vi "Config_flotas_baja_velocidad.vi"(11 "file path (dialog if empty)":path) -> (0 "Radios ruedas":dbl[](array[numeric]), 1 "Distancias generales":dbl[](array[numeric]), 2 "Puntos medios de las ventanas":dbl[][](array[numeric]), 3 "Distancia de acelerómetros":dbl[](array[numeric]), 5 "Distacias y medidas de dispositivos":bool=TRUE, 7 "Series_flota":string[](array[string]))   [LabVIEW 2015]
panel:
  out "text":string
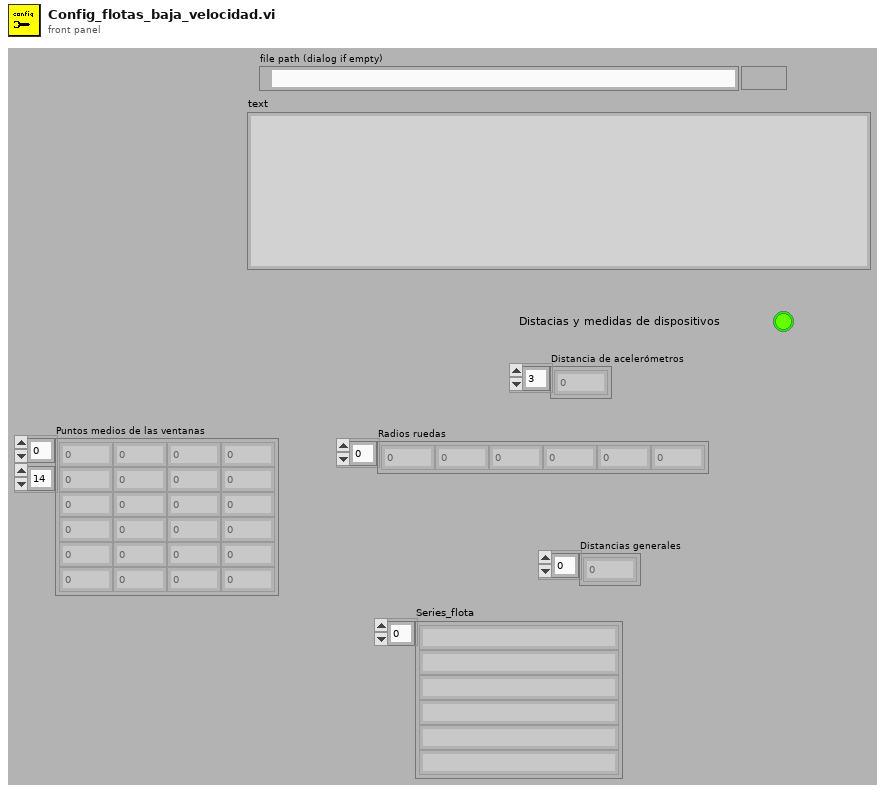
[diagram p1: front panel]
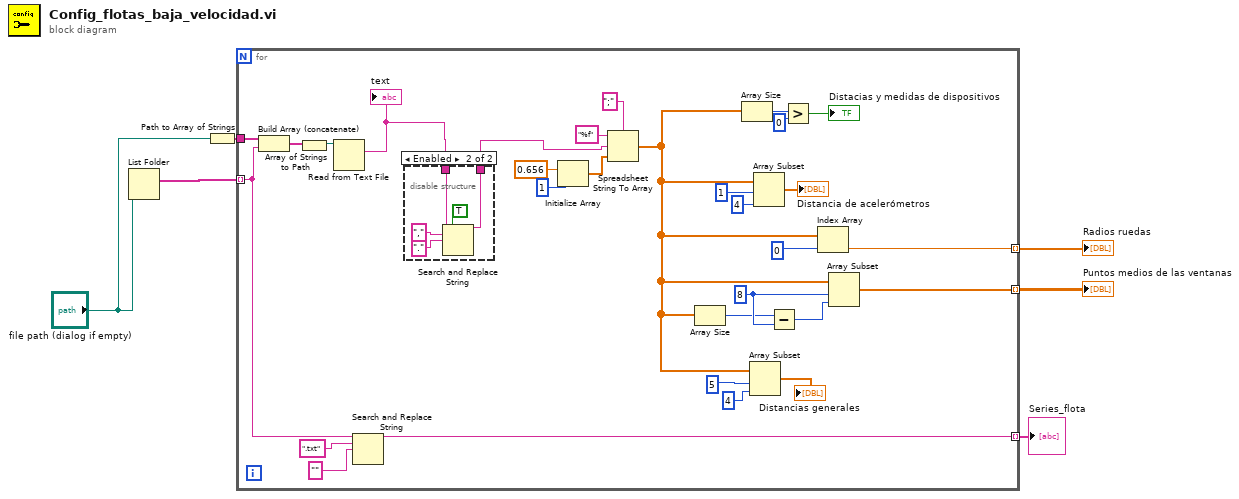
[diagram p0: block diagram]
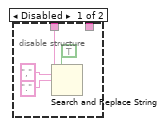
[diagram p2: hidden frame]
diagram:
  n1 = List Folder(path="file path (dialog if empty)") -> (filenames=w4:string[])  [unwired: 3 in, 3 out]
  n2 = Path to Array of Strings(0:"file path (dialog if empty)") -> (2:w5:string[])  [unwired: 1 out]
  n3 = for {
    tunnel: w5 -> [w20]
    tunnel: w4 -> [w14] mode=indexing
    tunnel: [w17] -> w3 mode=indexing
    tunnel: [w13] -> w2 mode=indexing
    tunnel: [w10] -> w1 mode=indexing
    w25 = 8 ("index")
    n4 = Build Array (concatenate)(w20, w14) -> (w19:string[])
    n5 = Array of Strings to Path(0:w19) -> (2:w18:path)  [unwired: 1 out]
    n6 = Read from Text File(file (use dialog)=w18) -> (text=w8:string)  [unwired: 3 in, 3 out]
    "text" <- w8
    n7 = Search and Replace String(input string=w14, search string=".txt" ("substring (\"\")"), replace string="" ("substring (\"\")")) -> (result string=w13:string)  [unwired: 5 in, 3 out]
    n8 = disable-structure shown="Enabled" {
      disable-tunnel: w8 -> [w37 w42]
      disable-tunnel: [_ w41] -> w7
      frame Disabled {
        n9 = Search and Replace String(replace all?=TRUE ("replace all? (F)"), input string=w37, search string=",", replace string="." ("replace string (\"\")")) -> ()  [unwired: 4 in, 4 out]
      }
      frame Enabled {
        n10 = Search and Replace String(replace all?=TRUE ("replace all? (F)"), input string=w42, search string=",", replace string="." ("replace string (\"\")")) -> (result string=w41:string)  [unwired: 4 in, 3 out]
      }
    }
    n11 = Initialize Array(0.656 ("element"), 1 ("dimension size")) -> (w33:dbl[])
    n12 = Spreadsheet String To Array(delimiter (Tab)=";" ("prompt (Open existing file)"), format string="%f", spreadsheet string=w7, array type (2D Dbl)=w33) -> (array=w11:dbl[])
    n13 = Array Size(array=w11) -> (size(s)=w24:i32)
    n14 = Array Size(array=w11) -> (size(s)=w32:i32)
    n15 = Array Subset(array=w11, index=5, length=4) -> (→"Distancias generales":dbl[])
    n16 = Array Subset(array=w11, index=1, length=4) -> (→"Distancia de acelerómetros":dbl[])
    n17 = Subtract(x=w24, y=w25) -> (x-y=w26:i32)
    n18 = Greater?(x=w32, y=0) -> (0:→"Distacias y medidas de dispositivos":bool)
    n19 = Index Array(array=w11, index=0) -> (element=w10:dbl)
    n20 = Array Subset(array=w11, index=w25, length=w26) -> (w17:dbl[])
  }
  "Puntos medios de las ventanas" <- w3
  "Series_flota" <- w2
  "Radios ruedas" <- w1
